vi "Main.vi"(10 "ACQ SUBPANE":refnum<vi>, 11 "Module Admin":refnum<class "Delacor_lib_QMH_Module Admin.lvclass">) -> ()   [LabVIEW 2019, in "ACQUISITION.lvlib"]
doc: "This template is based off of the Queued Message Handler design pattern and the Queued Message Handler project template that ships with LabVIEW.\n\nThe main difference is that the queue is private to this module and communication between modules is performed via Broadcast and Request events.\n\nRequest events are wrapped in public API methods and are handled in the Event Handling Loop (EHL) of this VI. Any module can register for Broadcast events sent by this module. The EHL generates messages based on user interface actions.\n\nThe Message Handling Loop (MHL) processes messages generated by the EHL, or by other messages. The messages are string values, so new messages can be added easily to the Message Cases case structure in the MHL. Each message cluster can also provide an optional value for Message Data, which is a variant that can be converted to whatever message-specific data is required.\n_____\nBased on Delacor QMH Project Template 5.0.0.82."
uses:
  ACQUISITION.lvlib
  <vilib>/Delacor/Delacor QMH/Libraries/Module Admin_class/Delacor_lib_QMH_Module Admin.lvclass
  Module Data--cluster.ctl
  STOP HELPER LOOP ACQ Argument--cluster.ctl
  <vilib>/Delacor/Delacor QMH/Libraries/Message Queue_class/Delacor_lib_QMH_Message Queue.lvclass/Delacor_lib_QMH_Message Queue.ctl
  Stop Argument--cluster.ctl
  <vilib>/Delacor/Delacor QMH/Libraries/Module Admin_class/Delacor_lib_QMH_Module Admin.lvclass/Delacor_lib_QMH_Module Admin.ctl
  <vilib>/Utility/miscctls.llb/LVPointTypeDef.ctl
  <vilib>/Delacor/Delacor QMH/Libraries/Message Queue_class/Delacor_lib_QMH_Enqueue Message (Single).vi
  <vilib>/Delacor/Delacor QMH/Libraries/Module Admin_class/Delacor_lib_QMH_Get External Launch.vi
  <vilib>/Utility/error.llb/Error Cluster From Error Code.vi
  <vilib>/ErrorRing/Error Ring.xnode
  <vilib>/Delacor/Delacor QMH/Libraries/Message Queue_class/Delacor_lib_QMH_Message Queue.lvclass
  ANALISIS/ANALISIS .lvlib
panel:
  out "Tanque":dbl(slide) scale=0.0..1.0
  out "Porcentaje de agua en el tanque":dbl
  in  "Iniciar adquisición":bool
  in  "Simulate MHL Error":bool
  in  "Simulate EHL Error":bool
  out "error out":errorcluster
  out "Status":string
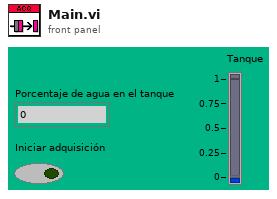
[diagram p1: front panel]
types:
  T1 = typedef "ACQUISITION.lvlib/Request Events--cluster.ctl" = cluster{"Stop Module":refnum<user-event>, "Show Panel":refnum<user-event>, "Hide Panel":refnum<user-event>, "Get Module Execution Status":refnum<user-event>, "Show Diagram":refnum<user-event>, "START HELPER LOOP ACQ":refnum<user-event>, "STOP HELPER LOOP ACQ":refnum<user-event>}
  T2 = typedef "ACQUISITION.lvlib/Module Data--cluster.ctl" = cluster{"Status":string}
  T3 = typedef "ACQUISITION.lvlib/STOP HELPER LOOP ACQ Argument--cluster.ctl" = cluster{"Boolean":bool}
  T4 = enum32{"invalid lock state", "Not Locked", "Locked (No Password)", "Password-protected"}
  T5 = typedef "ACQUISITION.lvlib/Stop Argument--cluster.ctl" = cluster{"Origin":string, "Exit via Stop Module Req?":bool, "Wait for Module to stop?":bool}
  T6 = typedef "LVPointTypeDef.ctl" = cluster{"Horizontal":i16, "Vertical":i16}
  T7 = enum32{"Invalid", "Standard", "Closed", "Hidden", "Minimized", "Maximized"}
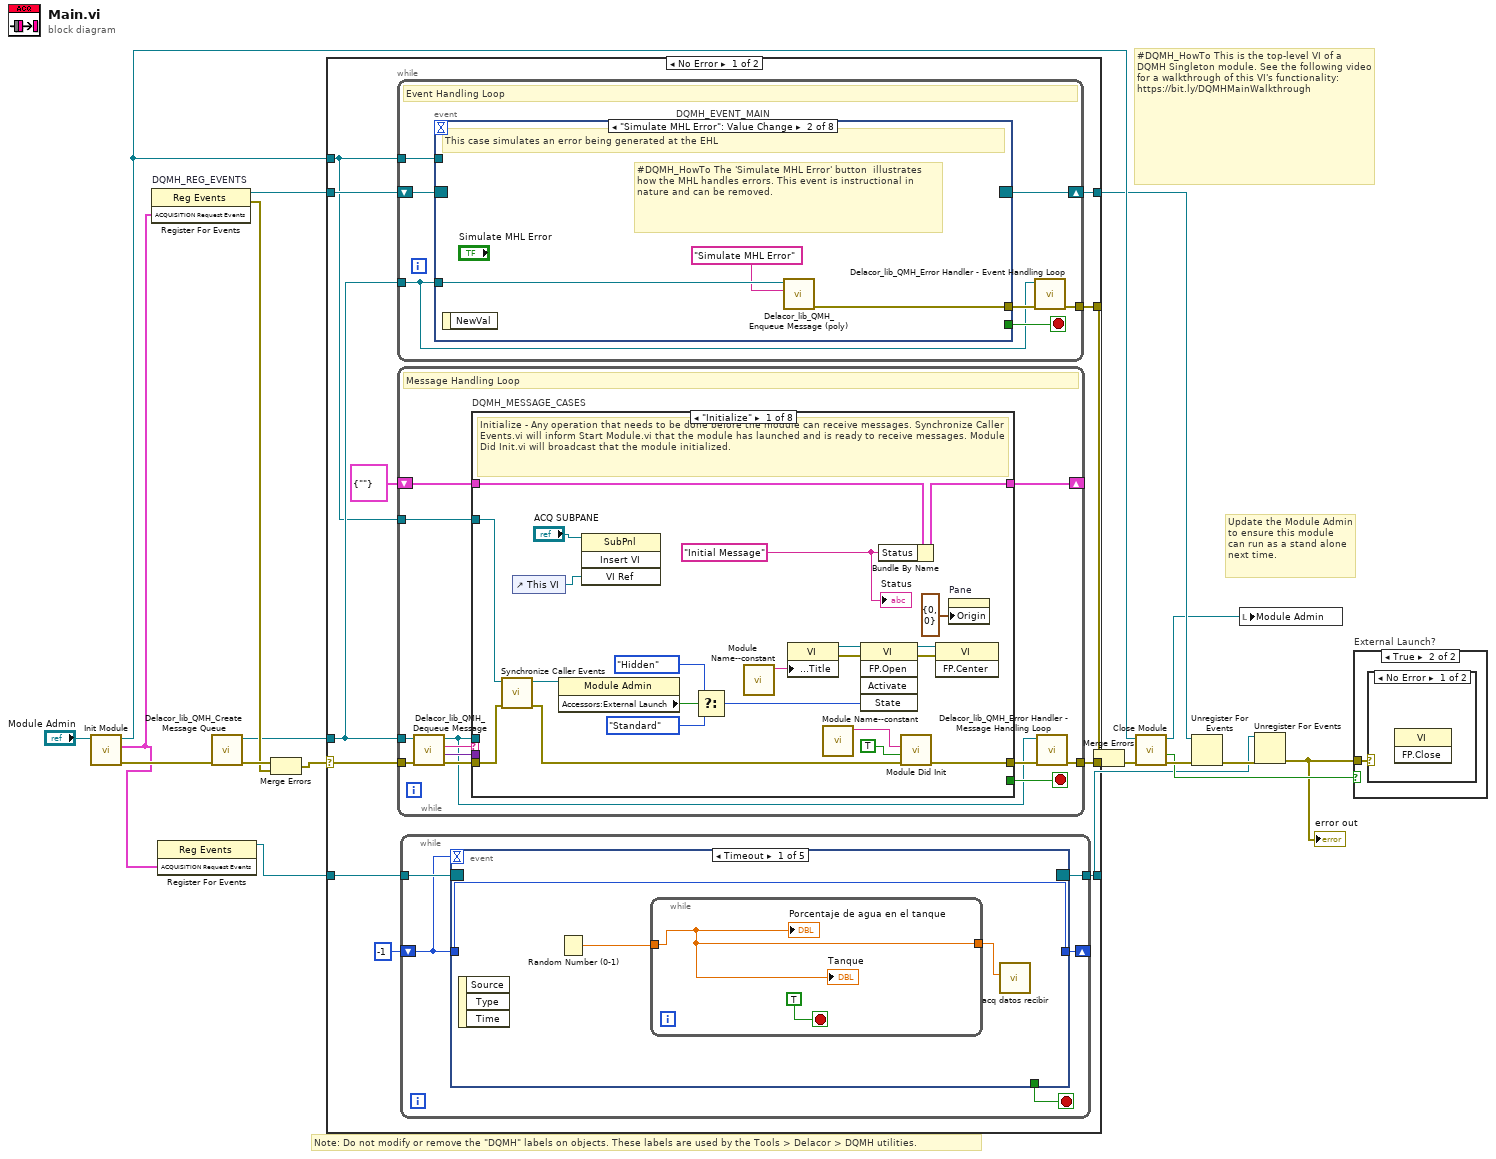
[diagram p0: block diagram]
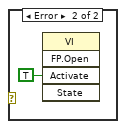
[diagram p3: hidden frame]
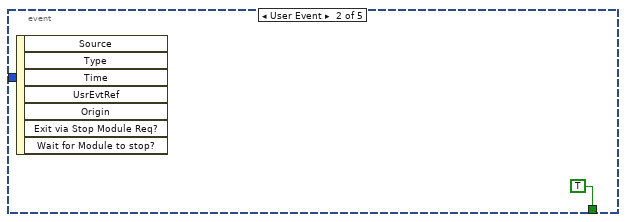
[diagram p4: hidden frame]
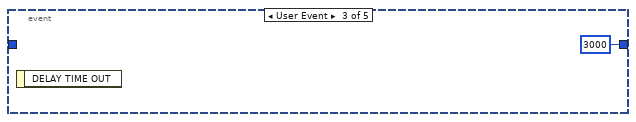
[diagram p5: hidden frame]
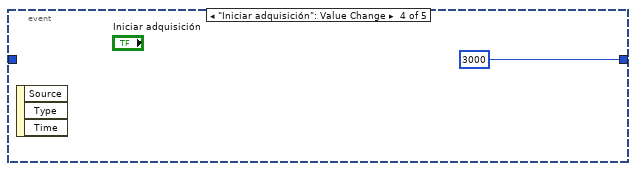
[diagram p6: hidden frame]
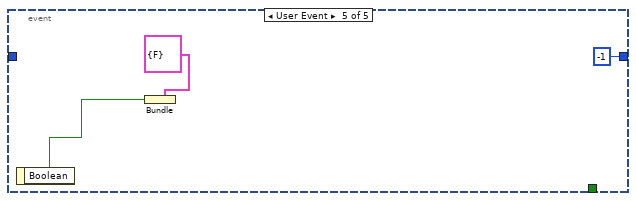
[diagram p7: hidden frame]
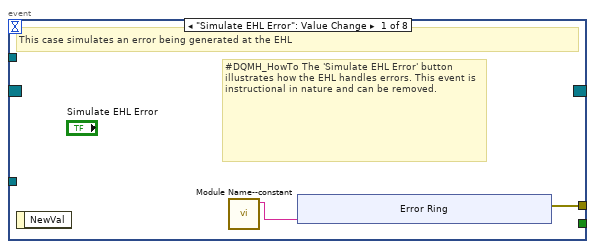
[diagram p8: hidden frame]
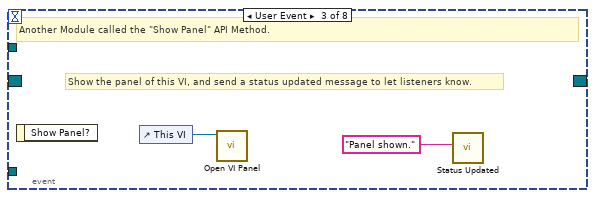
[diagram p9: hidden frame]
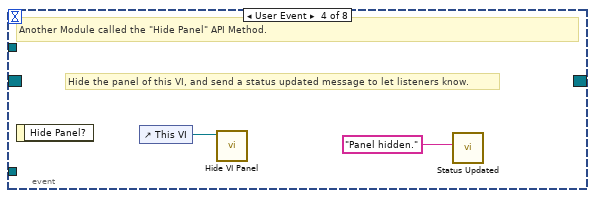
[diagram p10: hidden frame]
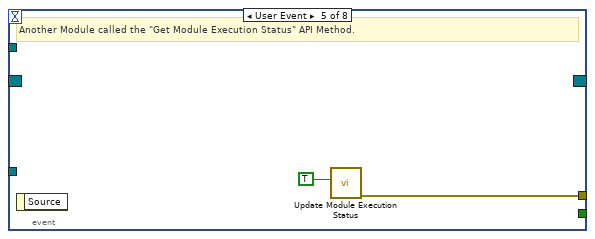
[diagram p11: hidden frame]
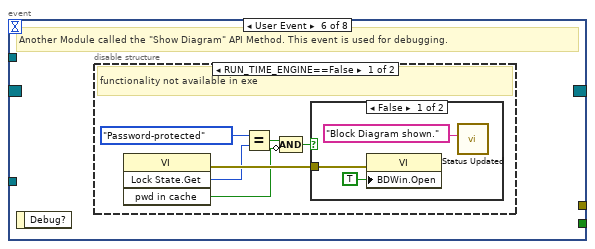
[diagram p12: hidden frame]
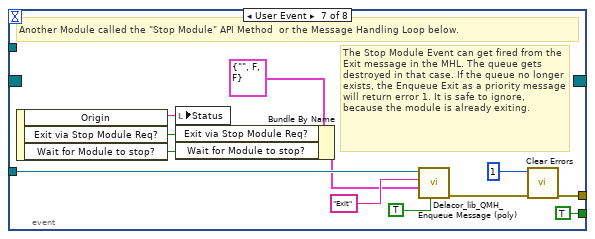
[diagram p15: hidden frame]
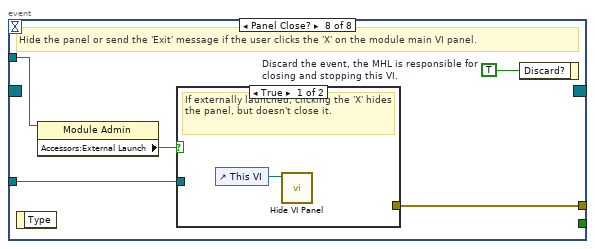
[diagram p16: hidden frame]
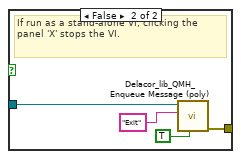
[diagram p17: hidden frame]
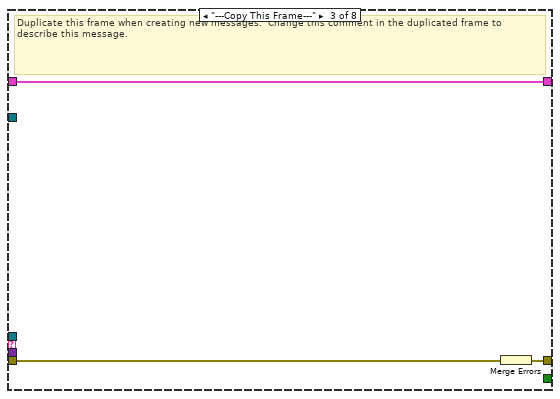
[diagram p19: hidden frame]
diagram:
  # "#DQMH_HowTo This is the top-level VI of a DQMH Singleton module. See the following video for a walkthrough of this VI's functionality: https://bit.ly/DQMHMainWalkthrough"
  # "Note: Do not modify or remove the \"DQMH\" labels on objects. These labels are used by the Tools > Delacor > DQMH utilities."
  # "Update the Module Admin to ensure this module can run as a stand alone next time."
  n1 = call "Init Module.vi"("Singleton Module Admin in"="Module Admin") -> ("error out"=w19:errorcluster, "ACQUISITION Request Events"=w5:T1, "Singleton Module Admin out"=w12:refnum<class "Delacor_lib_QMH_Module Admin.lvclass">)  [unwired: 8 in]
  n2 = register-events "DQMH_REG_EVENTS"(w5) -> (reference out=w10:refnum<event-registration>, error out=w13:errorcluster)  [unwired: 2 in]
  n3 = register-events(w5) -> (reference out=w4:refnum<event-registration>)  [unwired: 2 in, 1 out]
  n4 = call <vilib>:"Delacor_lib_QMH_Create Message Queue.vi"("error in (no error)"=w19) -> ("error out"=w15:errorcluster, "Message Queue"=w9:refnum<class "Delacor_lib_QMH_Message Queue.lvclass">)  [unwired: 9 in]
  n5 = Merge Errors(w15, w13) -> (w14:errorcluster)
  n6 = case shown="No Error" w14 {
    selector: w14 -> [w29 w206]
    tunnel: [w31 w205] -> w20
    tunnel: [w28 w211] -> w11
    tunnel: w10 -> [w26 w211]
    tunnel: w9 -> [w25 w204]
    tunnel: [w30 _] -> w17
    tunnel: w12 -> [w24 w207]
    tunnel: w4 -> [w23 w203]
    tunnel: [w22 w203] -> w2
    frame No Error {
      n7 = while {
        tunnel: w25 -> [w48]
        shift-right: [w51] -> w28
        shift-left: w26 -> [w52]
        tunnel: [w53] -> w30
        tunnel: w24 -> [w49]
        stop <- w50 stop-if-true
        # "Event Handling Loop"
        n8 = event "DQMH_EVENT_MAIN" shown="[1] \"Simulate MHL Error\": Value Change" {
          selector: w52 -> [_ _ _ _ _ _ _ _]
          dyn-events: [_ _ _ _ _ _ _ _] -> w51
          timeout: _ -> [_ _ _ _ _ _ _ _]
          tunnel: [_ _ _ _ _ _ TRUE ("Discard?") _] -> w50
          tunnel: w48 -> [_ w65 _ _ _ _ w89 w96]
          tunnel: [w56 w66 _ _ w72 _ w92 w98] -> w54
          tunnel: w49 -> [_ _ _ _ _ _ _ w95]
          event "Simulate EHL Error": Value Change {
            # "#DQMH_HowTo The 'Simulate EHL Error' button  illustrates how the EHL handles errors. This event is instructional in nature and can be removed."
            # "This case simulates an error being generated at the EHL"
            n9 = event-data() -> ()  [unwired: 1 in, 1 out]
            n10 = call "Module Name--constant.vi"() -> ("Module Name"=w55:string)  [unwired: 11 in]
            n11 = xnode "Error Ring"("parameter 0"=w55) -> ("error out"=w56:errorcluster)
          }
          event "Simulate MHL Error": Value Change {
            # "#DQMH_HowTo The 'Simulate MHL Error' button  illustrates how the MHL handles errors. This event is instructional in nature and can be removed."
            # "This case simulates an error being generated at the EHL"
            n12 = event-data() -> ()  [unwired: 1 in, 1 out]
            n13 = call-poly <vilib>:"Delacor_lib_QMH_Enqueue Message (poly).vi"("Message"="Simulate MHL Error", "Message Queue in"=w65) -> ("error out"=w66:errorcluster)  [unwired: 8 in, 1 out]
          }
          event User Event {
            # "Show the panel of this VI, and send a status updated message to let listeners know."
            # "Another Module called the \"Show Panel\" API Method."
            n14 = event-data() -> ()  [unwired: 1 in, 1 out]
            n15 = control-ref of="This VI"() -> (w68:refnum<vi>)
            n16 = call "Open VI Panel.vi"("VI"=w68) -> ()  [unwired: 10 in, 1 out]
            n17 = call "Status Updated.vi"("Status"="Panel shown." ("format string")) -> ()  [unwired: 10 in, 1 out]
          }
          event User Event {
            # "Hide the panel of this VI, and send a status updated message to let listeners know."
            # "Another Module called the \"Hide Panel\" API Method."
            n18 = event-data() -> ()  [unwired: 1 in, 1 out]
            n19 = control-ref of="This VI"() -> (w70:refnum<vi>)
            n20 = call "Hide VI Panel.vi"("VI"=w70) -> ()  [unwired: 10 in, 1 out]
            n21 = call "Status Updated.vi"("Status"="Panel hidden." ("format string")) -> ()  [unwired: 10 in, 1 out]
          }
          event User Event {
            # "Another Module called the \"Get Module Execution Status\" API Method."
            n22 = event-data() -> ()  [unwired: 1 in, 1 out]
            n23 = call "Update Module Execution Status.vi"("Running?"=TRUE) -> ("error out"=w72:errorcluster)  [unwired: 10 in]
          }
          event User Event {
            # "Another Module called the \"Show Diagram\" API Method. This event is used for debugging."
            n24 = event-data() -> ()  [unwired: 1 in, 1 out]
            n25 = disable-structure shown="RUN_TIME_ENGINE==False" {
              frame condition #0 (active) {
                # "functionality not available in exe"
                n26 = invoke class="VI" method="Lock State.Get"() -> (error out=w78:errorcluster, "Get Lock State"=w77:T4, "pwd in cache"=w74:bool)  [unwired: 4 in, 1 out]
                n27 = Equal?(x=T4."Password-protected", y=w77) -> (x = y?=w75:bool)
                n28 = Compound Arithmetic op=AND(w75, invert w74) -> (w73:bool)
                n29 = case shown="False" w73 {
                  tunnel: w78 -> [w81 _]
                  frame False {
                    n30 = property class="VI"(error in=w81, "BDWin.Open"=TRUE ("Block Diagram Window:Open")) -> ()  [unwired: 1 in, 2 out]
                    n31 = call "Status Updated.vi"("Status"="Block Diagram shown." ("format string")) -> ()  [unwired: 10 in, 1 out]
                  }
                  frame True {
                    # "Password-protected VI, and the password is not in the cache. Do not show the diagram."
                  }
                }
              }
              frame condition #1 {
              }
            }
          }
          event User Event {
            # "The Stop Module Event can get fired from the Exit message in the MHL. The queue gets destroyed in that case. If the queue no longer exists, the Enqueue Exit as a priority message will return error 1. It is safe to ignore, because the module is already exiting."
            # "Another Module called the \"Stop Module\" API Method  or the Message Handling Loop below."
            n32 = event-data() -> ("Origin"=w88:string, "Exit via Stop Module Req?"=w84:bool, "Wait for Module to stop?"=w83:bool)  [unwired: 1 in]
            n33 = local write "Status"(w88) -> ()
            n34 = Bundle By Name(cluster=T5 {"Origin"="", "Exit via Stop Module Req?"=FALSE, "Wait for Module to stop?"=FALSE} ("Stop Argument"), "Exit via Stop Module Req?"=w84, "Wait for Module to stop?"=w83) -> (w82:T5)
            n35 = call-poly <vilib>:"Delacor_lib_QMH_Enqueue Message (poly).vi"("Priority Message? (F)"=TRUE, "Message Data"=w82, "Message"="Exit", "Message Queue in"=w89) -> ("error out"=w93:errorcluster)  [unwired: 6 in, 1 out]
            n36 = call <vilib>:"Clear Errors.vi"("error in (no error)"=w93, "specific error code to clear (0: all)"=1) -> ("error out"=w92:errorcluster)  [unwired: 4 in, 1 out]
          }
          event Panel Close? {
            w97 = TRUE  # Discard the event, the MHL is responsible for closing and stopping this VI.
            # "Hide the panel or send the 'Exit' message if the user clicks the 'X' on the module main VI panel."
            n37 = event-data() -> ()  [unwired: 1 in, 1 out]
            n38 = property class="Module Admin"(reference=w95) -> ("Accessors:External Launch"=w94:bool)  [unwired: 1 in, 2 out]
            n39 = case shown="True" w94 {
              tunnel: w96 -> [_ w102]
              tunnel: [_ w103] -> w98
              frame True {
                # "If externally launched, clicking the 'X' hides the panel, but doesn't close it."
                n40 = control-ref of="This VI"() -> (w99:refnum<vi>)
                n41 = call "Hide VI Panel.vi"("VI"=w99) -> ()  [unwired: 10 in, 1 out]
              }
              frame False {
                # "If run as a stand-alone VI, clicking the panel 'X' stops the VI."
                n42 = call-poly <vilib>:"Delacor_lib_QMH_Enqueue Message (poly).vi"("Priority Message? (F)"=TRUE, "Message"="Exit", "Message Queue in"=w102) -> ("error out"=w103:errorcluster)  [unwired: 7 in, 1 out]
              }
            }
            n43 = event-data("Discard?"=w97) -> ()  [unwired: 1 in, 1 out]
          }
        }
        n44 = call-dynamic "Delacor_lib_QMH_Error Handler - Event Handling Loop.vi"("error in (no error)"=w54, "Message Queue in"=w48) -> ("dup error in"=w53:errorcluster)  [unwired: 8 in, 1 out]
      }
      n45 = while {
        tunnel: w25 -> [w106]
        shift-right: [w110] -> _
        shift-left: T2 {"Status"=""} ("Data Cluster") -> [w111]
        tunnel: w29 -> [w114]
        tunnel: [w112] -> w31
        tunnel: w24 -> [w104]
        stop <- w109 stop-if-true
        # "Message Handling Loop"
        n46 = call-dynamic "Delacor_lib_QMH_Dequeue Message.vi"("error in (no error)"=w114, "Message Queue in"=w106) -> ("error out"=w113:errorcluster, "Message Data"=w107:variant, "Message"=w108:string, "Message Queue out"=w105:refnum<class "Delacor_lib_QMH_Message Queue.lvclass">)  [unwired: 6 in]
        n47 = case "DQMH_MESSAGE_CASES" shown="\"Initialize\"" w108 {
          selector: w108 -> [_ _ _ _ _ _ _ w190]
          tunnel: w105 -> [_ _ _ _ _ w160 w182 _]
          tunnel: w113 -> [w135 w139 w142 w144 w149 w167 w188 w192]
          tunnel: [w133 w139 w141 w144 w148 w163 w185 w193] -> w115
          tunnel: w111 -> [w124 w138 w140 w143 w146 w162 w181 w191]
          tunnel: [w123 w138 w140 w143 w146 w162 w181 w191] -> w110
          tunnel: [_ _ _ _ _ _ w180 _] -> w109
          tunnel: w107 -> [_ _ _ _ _ w161 w179 _]
          tunnel: w104 -> [w125 _ _ _ _ w159 w174 _]
          frame "Initialize" {
            w118 = "Initial Message" ("Initial Message")
            # "Initialize - Any operation that needs to be done before the module can receive messages. Synchronize Caller Events.vi will inform Start Module.vi that the module has launched and is ready to receive messages. Module Did Init.vi will broadcast that the module initialized."
            n48 = call "Synchronize Caller Events.vi"("error in (no error)"=w135, "Singleton Module Admin in"=w125) -> ("error out"=w134:errorcluster, "Singleton Module Admin out"=w120:refnum<class "Delacor_lib_QMH_Module Admin.lvclass">)  [unwired: 8 in]
            n49 = control-ref of="This VI"() -> (w116:refnum<vi>)
            n50 = property class="Module Admin"(reference=w120) -> ("Accessors:External Launch"=w129:bool)  [unwired: 1 in, 2 out]
            n51 = invoke class="SubPnl" method="Insert VI"(reference="ACQ SUBPANE", "VI Ref"=w116) -> ()  [unwired: 2 in, 4 out]
            n52 = Select(t=T7."Hidden" ("State"), s=w129, f=T7."Standard" ("State")) -> (s? t:f=w126:T7)
            n53 = call "Module Name--constant.vi"() -> ("Module Name"=w132:string)  [unwired: 11 in]
            n54 = property class="VI"("Front Panel.Title"=w132) -> (reference out=w131:refnum<vi>, error out=w137:errorcluster)  [unwired: 2 in]
            n55 = call "Module Name--constant.vi"() -> ("Module Name"=w121:string)  [unwired: 11 in]
            n56 = invoke class="VI" method="FP.Open"(reference=w131, error in=w137, "State"=w126) -> (reference out=w130:refnum<vi>, error out=w136:errorcluster)  [unwired: 2 in, 3 out]
            n57 = Bundle By Name(cluster=w124, "Status"=w118) -> (w123:T2)
            n58 = call "Module Did Init.vi"("error in (no error)"=w134, "Initialized?"=TRUE, "Origin"=w121) -> ("error out"=w133:errorcluster)  [unwired: 8 in]
            n59 = invoke class="VI" method="FP.Center"(reference=w130, error in=w136) -> ()  [unwired: 1 in, 3 out]
            n60 = property on="Pane" class="Pane"("Origin"=T6 {"Horizontal"=0, "Vertical"=0}) -> ()  [unwired: 2 in, 2 out]
            "Status" <- w118
          }
          frame "--- Module Specific ---" {
            # "Separator -- The following cases handle messages specific to this Module."
          }
          frame "---Copy This Frame---" {
            # "Duplicate this frame when creating new messages.  Change this comment in the duplicated frame to describe this message."
            n61 = Merge Errors(w142) -> (w141:errorcluster)
          }
          frame "--- Exit and Error Handling---" {
            # "Separator - The following cases handle errors and exit messages."
          }
          frame "Simulate MHL Error" {
            # "#DQMH_HowTo The 'Simulate MHL Error' button  illustrates how the MHL handles errors. This event is instructional in nature and can be removed."
            # "Simulate an error occurring at the MHL"
            n62 = call "Module Name--constant.vi"() -> ("Module Name"=w145:string)  [unwired: 11 in]
            n63 = xnode "Error Ring"("parameter 0"=w145) -> ("error out"=w147:errorcluster)
            n64 = Merge Errors(w149, w147) -> (w148:errorcluster)
          }
          frame "Error" {
            # "#CodeRecommended - If you ever change the name of this \"Error\" message, you'll need to update the name in the Check Loop Error.vi as well."
            # "#CodeRecommended - If the module is running in standalone mode (External Launch = FALSE), this code will pop up an error dialog and call the 'Exit' message if an error occurs. Add more fine-grained error handling here."
            # "Error - Check the error message data and respond accordingly. This message is sent by the \"Error Handler\" VIs at the end of each loop in this application."
            n65 = property class="Module Admin"(reference=w159) -> ("Accessors:External Launch"=w158:bool)  [unwired: 1 in, 2 out]
            n66 = Variant To Data(error in=w167, type=errorcluster {"status"=FALSE, "code"=0, "source"=""} ("error constant"), Variant=w161) -> (data=w168:errorcluster, error out=w165:errorcluster)
            n67 = call "Module Name--constant.vi"() -> ("Module Name"=w157:string)  [unwired: 11 in]
            n68 = call "Error Reported.vi"("Additional Information"=w157, "Error"=w168) -> ()  [unwired: 9 in, 1 out]
            n69 = case shown="False" w158 {
              tunnel: [w173 _] -> w164
              tunnel: w160 -> [w171 _]
              tunnel: w168 -> [w172 _]
              frame False {
                # "If the module is running standalone, then pop up an error dialog and call the \"Exit\" message."
                n70 = call <vilib>:"Simple Error Handler.vi"("error in (no error)"=w172) -> ()  [unwired: 4 in, 5 out]
                n71 = call-poly <vilib>:"Delacor_lib_QMH_Enqueue Message (poly).vi"("Priority Message? (F)"=TRUE, "Message"="Exit", "Message Queue in"=w171) -> ("error out"=w173:errorcluster)  [unwired: 7 in, 1 out]
              }
              frame True {
                # "If the module was launched externally, calling the Error Reported broadcast VI is the only action performed by the \"Error\" message. The module's caller can then process the error appropriately."
              }
            }
            n72 = Merge Errors(w165, w164) -> (w163:errorcluster)
            n73 = local write "error out"(w163) -> ()
          }
          frame "Exit" {
            w178 = 91  # 91: not all Exit messages will have an argument
            w180 = TRUE  # Stop the VI
            # "Release the message queue reference"
            # "#CodeNeeded - Add any required cleanup code here"
            # "Exit - Exit the application."
            n74 = Variant To Data(error in=w188, type=T5 {"Origin"="", "Exit via Stop Module Req?"=FALSE, "Wait for Module to stop?"=FALSE} ("Stop Argument"), Variant=w179) -> (data=w176:T5, error out=w184:errorcluster)
            n75 = call <vilib>:"Clear Errors.vi"("error in (no error)"=w184, "specific error code to clear (0: all)"=w178) -> ("error out"=w187:errorcluster)  [unwired: 4 in, 1 out]
            n76 = control-ref of="This VI"() -> (w175:refnum<vi>)
            n77 = call-dynamic "Delacor_lib_QMH_Release Message Queue.vi"("error in (no error)"=w187, "Message Queue"=w182) -> ("error out"=w186:errorcluster)  [unwired: 9 in]
            n78 = call "Handle Exit.vi"("Stop Argument"=w176, "Admin in"=w174, "VI reference"=w175) -> ("error out"=w183:errorcluster)  [unwired: 7 in, 1 out]
            n79 = Merge Errors(w186, w183) -> (w185:errorcluster)
          }
          frame Default {
            # "'Default' case only runs if there is a message that isn't defined in any of the other cases.  Output a programming error."
            n80 = call "Module Name--constant.vi"() -> ("Module Name"=w189:string)  [unwired: 11 in]
            n81 = xnode "Error Ring"("parameter 0"=w190, "parameter 1"=w189) -> ("error out"=w194:errorcluster)
            n82 = Merge Errors(w192, w194) -> (w193:errorcluster)
          }
        }
        n83 = call-dynamic "Delacor_lib_QMH_Error Handler - Message Handling Loop.vi"("error in (no error)"=w115, "Message Queue in"=w105) -> ("dup error in"=w112:errorcluster)  [unwired: 8 in, 1 out]
      }
      n84 = while {
        tunnel: w23 -> [w36]
        tunnel: [w35] -> w22
        shift-right: [w33] -> _
        shift-left: -1 ("DELAY TIME OUT") -> [w32]
        stop <- w34 stop-if-true
        n85 = event shown="[0] Timeout" {
          selector: w36 -> [_ _ _ _ _]
          dyn-events: [_ _ _ _ _] -> w35
          timeout: w32 -> [_ _ _ _ _]
          tunnel: [_ TRUE _ _ _] -> w34
          tunnel: [w39 _ 3000 ("DELAY TIME OUT") 3000 ("DELAY TIME OUT") -1 ("DELAY TIME OUT")] -> w33
          tunnel: w32 -> [w39 _ _ _ _]
          event Timeout {
            n86 = event-data() -> ()  [unwired: 1 in, 3 out]
            n87 = Random Number (0-1)() -> (number: 0 to 1=w38:dbl)
            n88 = while {
              tunnel: w38 -> [w40]
              tunnel: [w40] -> w37
              stop <- TRUE stop-if-true
              "Porcentaje de agua en el tanque" <- w40
              "Tanque" <- w40
            }
            n89 = call "acq datos recibir.vi"("Numeric"=w37) -> ()  [unwired: 10 in, 1 out]
          }
          event User Event {
            n90 = event-data() -> ()  [unwired: 1 in, 7 out]
          }
          event User Event {
            n91 = event-data() -> ()  [unwired: 1 in, 1 out]
          }
          event "Iniciar adquisición": Value Change {
            n92 = event-data() -> ()  [unwired: 1 in, 3 out]
          }
          event User Event {
            n93 = event-data() -> ("Boolean"=w47:bool)  [unwired: 1 in]
            n94 = Bundle(cluster=T3 {"Boolean"=FALSE} ("STOP HELPER LOOP ACQ Argument"), "Boolean"=w47) -> ()  [unwired: 1 out]
          }
        }
      }
    }
    frame Error {
      # "Synchronize Caller Events.vi will inform Start Module.vi that the module has launched and will let the code calling Start Module.vi register for broadcasts and would permit the caller receive the broadcast that an error occurred at launch time."
      n95 = call-dynamic "Delacor_lib_QMH_Release Message Queue.vi"("error in (no error)"=w206, "Message Queue"=w204) -> ("error out"=w205:errorcluster)  [unwired: 9 in]
      n96 = call "Synchronize Caller Events.vi"("Singleton Module Admin in"=w207) -> ("error out"=w212:errorcluster)  [unwired: 9 in, 1 out]
      n97 = call "Module Name--constant.vi"() -> ("Module Name"=w210:string)  [unwired: 11 in]
      n98 = Format Into String(format string="An error occurred during initialization. %s is no longer running.", w210) -> (resulting string=w208:string)  [unwired: 2 in, 1 out]
      n99 = Merge Errors(w205, w212) -> (w213:errorcluster)
      n100 = call "Error Reported.vi"("Additional Information"=w208, "Error"=w213) -> ()  [unwired: 9 in, 1 out]
    }
  }
  n101 = Merge Errors(w17, w20) -> (w16:errorcluster)
  n102 = call "Close Module.vi"("error in (no error)"=w16, "Module Admin in"=w12) -> ("error out"=w18:errorcluster, "External Launch"=w6:bool, "Module Admin out"=w7:refnum<class "Delacor_lib_QMH_Module Admin.lvclass">)  [unwired: 7 in]
  n103 = Unregister For Events(event registration refnum=w11, error in=w18) -> (error out=w3:errorcluster)
  n104 = local write "Module Admin"(w7) -> ()
  n105 = Unregister For Events(event registration refnum=w2, error in=w3) -> (error out=w1:errorcluster)
  "error out" <- w1
  n106 = case "External Launch?" shown="True" w6 {
    tunnel: w1 -> [_ w214]
    frame False {
    }
    frame True {
      n107 = case shown="No Error" w214 {
        frame No Error {
          n108 = invoke class="VI" method="FP.Close"() -> ()  [unwired: 3 in, 3 out]
        }
        frame Error {
          n109 = invoke class="VI" method="FP.Open"("Activate"=TRUE ("Activate?")) -> ()  [unwired: 4 in, 5 out]
        }
      }
    }
  }
